vi "CreateFakeTestListener.vi"(8 "error in (no error)":errorcluster) -> (0 "error out":errorcluster, 3 "FakeTestListener":refnum<class "FakeTestListener.lvclass">)   [LabVIEW 2019, in "TestResultTestSupport.lvlib" / "FakeTestListener.lvclass"]
uses:
  FakeTestListener.lvclass
  FakeTestListener.lvclass/FakeTestListener.ctl
panel:
  in  "FakeTestListener In":refnum<class "FakeTestListener.lvclass">
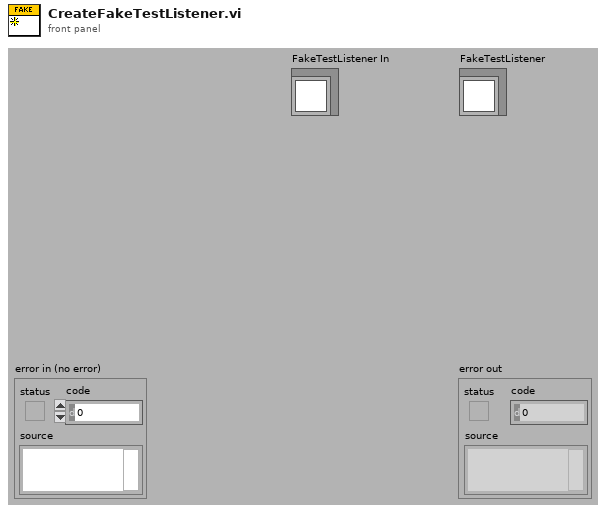
[diagram p1: front panel]
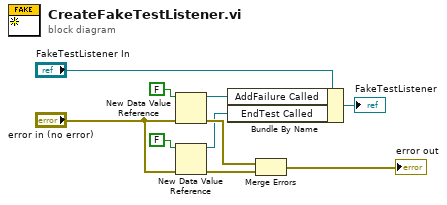
[diagram p0: block diagram]
diagram:
  n1 = New Data Value Reference(data value=FALSE, error in="error in (no error)") -> (data value reference=w8:refnum<data-value>, error out=w3:errorcluster)
  n2 = New Data Value Reference(data value=FALSE, error in="error in (no error)") -> (data value reference=w2:refnum<data-value>, error out=w4:errorcluster)
  n3 = Bundle By Name(cluster="FakeTestListener In", "AddFailure Called"=w8, "EndTest Called"=w2) -> (→"FakeTestListener":refnum<class "FakeTestListener.lvclass">)
  n4 = Merge Errors(w3, w4) -> (→"error out":errorcluster)
